vi "PrependRows_D.vi"(10 "Prepend Value":dbl, 11 "Input":dbl[][](array[numeric])) -> (3 "Output":dbl[][](array[numeric]))   [LabVIEW 2013]
doc: "This VI takes a 2D array, and prepends a value to each row."
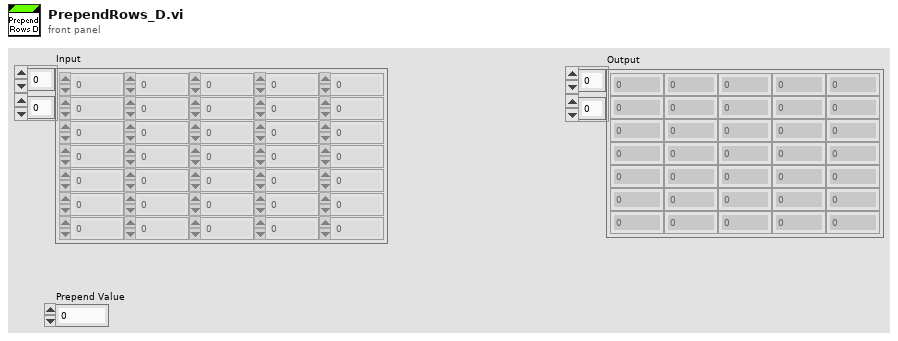
[diagram p1: front panel]
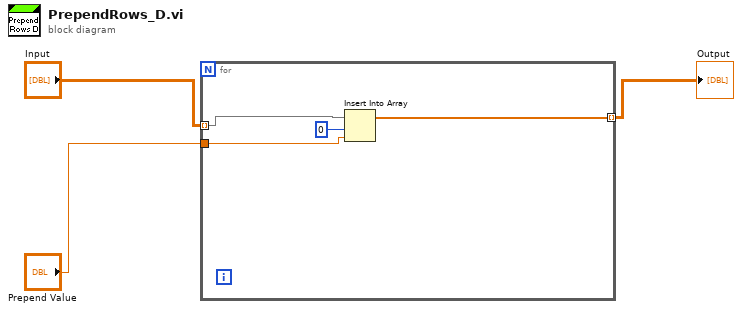
[diagram p0: block diagram]
diagram:
  n1 = for {
    tunnel: "Input" -> [w6] mode=indexing
    tunnel: [w5] -> w2 mode=indexing
    tunnel: "Prepend Value" -> [w4]
    n2 = Insert Into Array(array=w6, index=0, new element=w4) -> (w5:dbl[])
  }
  "Output" <- w2
